vi "camera_capture.vi"(11 "dup Message Queue":refnum<queue>) -> ()   [LabVIEW 2017]
uses:
  UI Error Handlers/support/Message Queue/Message Cluster.ctl
  <vilib>/userdefined/High Color/IMAQdx.ctl
  <vilib>/vision/Avi.llb/IMAQ AVI2 Codec Path.ctl
  Globals/Global - All RT Loop Stop.vi
  <vilib>/vision/driver/NI_Vision_Acquisition_Software.lvlib
  UI Error Handlers/support/Message Queue/Message Queue.lvlib
panel:
  out "concatenated string 2":string
  in  "Boolean":bool
  out "Codec Names":string[](array[string])
  in  "stop":bool
  out "Webcam":T1(plugin-control)
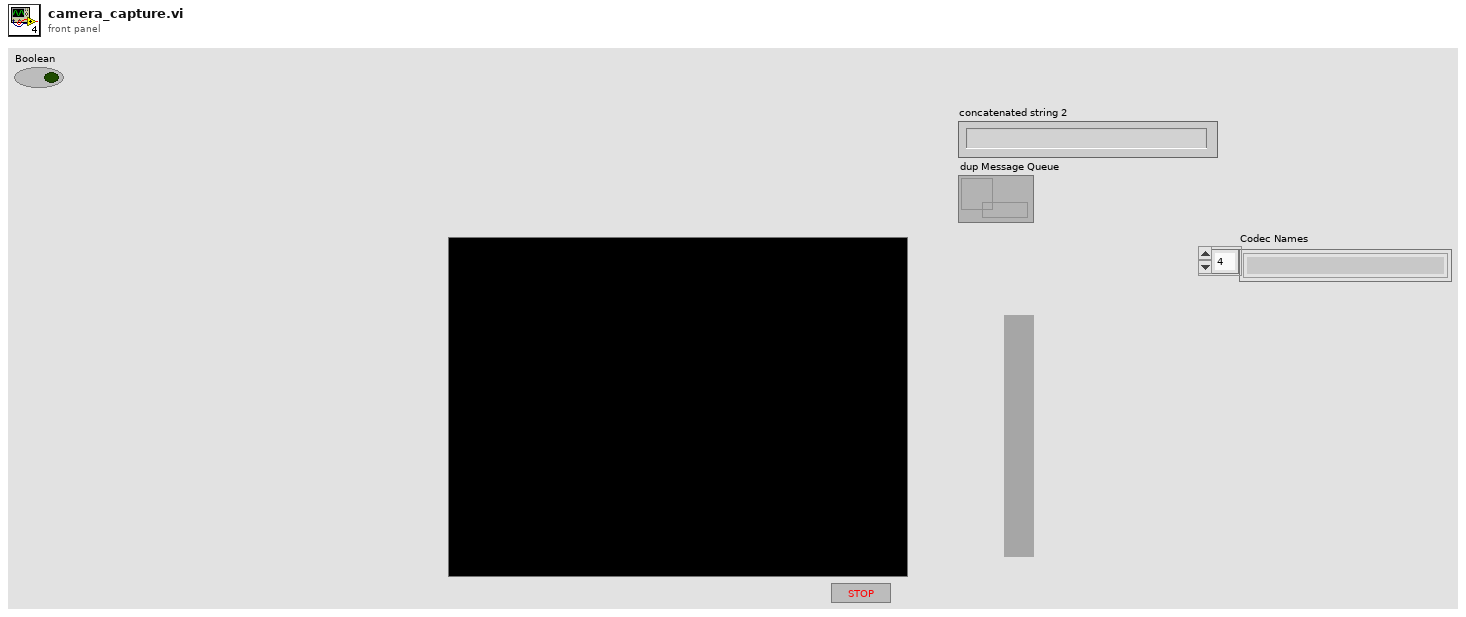
[diagram p1: front panel]
types:
  T1 = typedef "IMAQ Image.ctl" = refnum<image>
  T2 = typedef "IMAQdx.ctl" = refnum<k21>
  T3 = typedef "Image Type" = u32
  T4 = typedef "IMAQ AVI2 Refnum.ctl" = refnum<k20>
  T5 = typedef "IMAQ AVI2 Codec Path.ctl" = u32
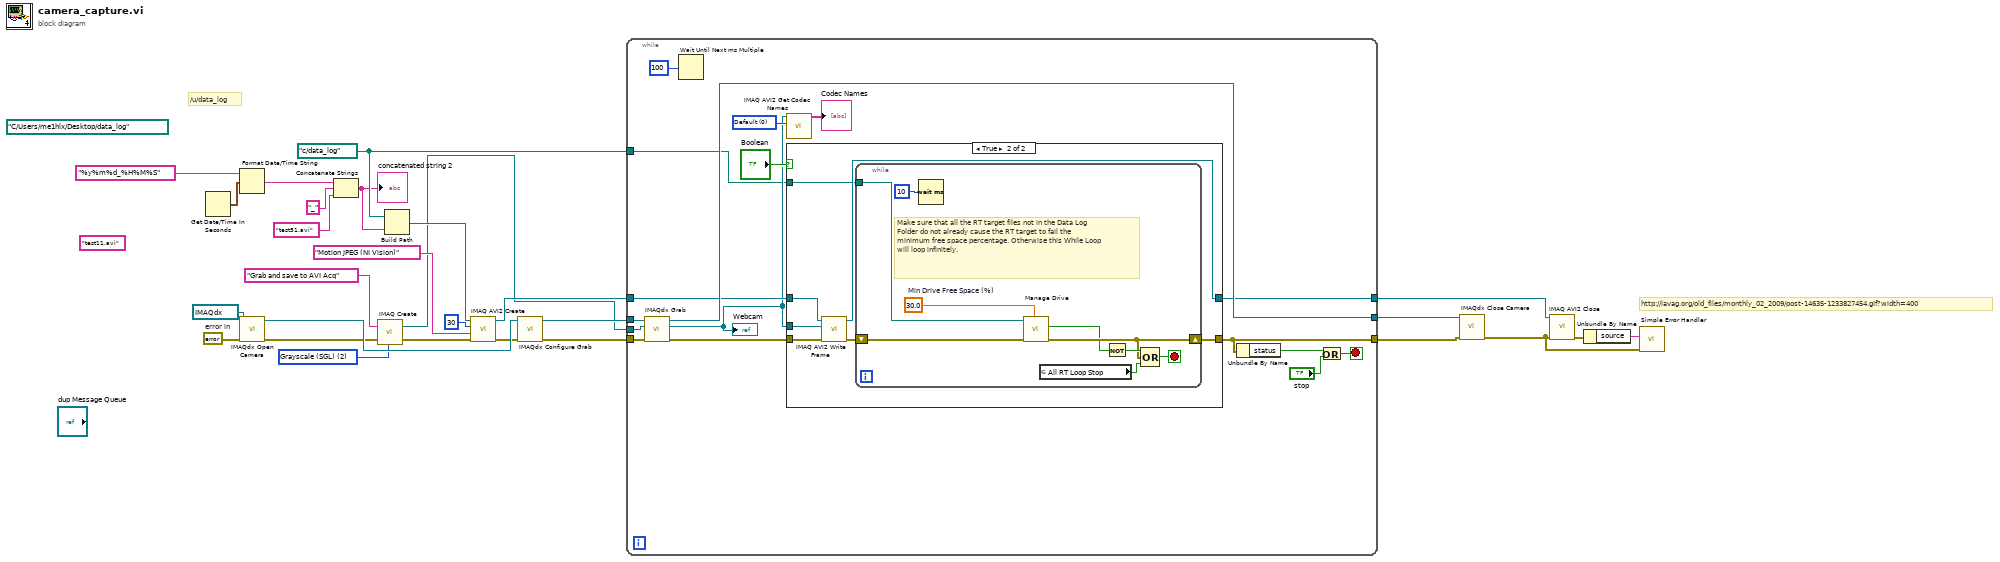
[diagram p0: block diagram]
diagram:
  (unwired) path "C:/Users/me1hlx/Desktop/data_log" ("AVI Path")
  (unwired) "test11.avi" ("name or relative path")
  w3 = path "c:/data_log" ("AVI Path")
  w17 = T3 2 items=["Grayscale (U8)", "Grayscale (I16)", "Grayscale (SGL)", "Complex (CSG)", "RGB (U32)", "HSL (U32)", "RGB (U64)", "Grayscale (U16)"] ("Image Type")
  w20 = errorcluster {"status"=FALSE, "code"=0, "source"=""}  # error in
  # "/u/data_log"
  # "http://lavag.org/old_files/monthly_02_2009/post-14635-1233827454.gif?width=400"
  n1 = Get Date/Time In Seconds() -> (seconds since 1Jan1904=w7:timestamp)
  n2 = Format Date/Time String(time format string (%c)="%y%m%d_%H%M%S", seconds (now)=w7) -> (date/time string=w6:string)  [unwired: 1 out]
  n3 = call <vilib>:"IMAQdx Open Camera.vi"("error in"=w20, "Session In"=T2 "cam0") -> ("error out"=w16:errorcluster, "Session Out"=w22:T2)  [unwired: 8 in]
  n4 = Concatenate Strings(w6, "_" ("string"), "test51.avi" ("name or relative path")) -> (w2:string)
  "concatenated string 2" <- w2
  n5 = call "IMAQ Create"("Image Name"="Grab and save to AVI Acq", "Image Type"=w17, "error in (no error)"=w16) -> ("New Image"=w9:T1, "error out"=w15:errorcluster)  [unwired: 2 in]
  n6 = Build Path(base path=w3, name or relative path=w2) -> (appended path=w19:path)
  n7 = call "IMAQ AVI2 Create"("error in (no error)"=w15, "Codec"="Motion JPEG (NI Vision)", "Frames Per Second"=u32 30, "AVI Path"=w19) -> ("error out"=w14:errorcluster, "AVI Refnum"=w12:T4)  [unwired: 6 in]
  n8 = call <vilib>:"IMAQdx Configure Grab.vi"("error in"=w14, "Session In"=w22) -> ("error out"=w10:errorcluster, "Session Out"=w11:T2)  [unwired: 8 in]
  n9 = while {
    tunnel: w10 -> [w45]
    tunnel: w11 -> [w44]
    tunnel: w9 -> [w43]
    tunnel: [w30] -> w28
    tunnel: [w42] -> w27
    tunnel: w12 -> [w34]
    tunnel: [w32] -> w23
    tunnel: w3 -> [w29]
    stop <- w38 stop-if-true
    w37 = T5 0 items=["Default", "System", "Built in Vision"] ("Codec Source")
    n10 = call <vilib>:"IMAQdx Grab.vi"("error in"=w45, "Image In"=w43, "Session In"=w44) -> ("error out"=w31:errorcluster, "Image Out"=w33:T1, "Session Out"=w42:T2)  [unwired: 5 in, 1 out]
    "Webcam" <- w33
    n11 = Wait Until Next ms Multiple(millisecond multiple=u32 100 ("milliseconds to wait")) -> ()  [unwired: 1 out]
    n12 = call "IMAQ AVI2 Get Codec Names"("Codec Source"=w37, "Image"=w33) -> ("Codec Names"=→"Codec Names":string[])  [unwired: 8 in, 1 out]
    n13 = case shown="True" "Boolean" {
      tunnel: w34 -> [w47 w54]
      tunnel: w33 -> [_ w53]
      tunnel: [w47 w52] -> w32
      tunnel: w31 -> [w46 w51]
      tunnel: [w46 w48] -> w30
      tunnel: w29 -> [_ w50]
      frame False {
      }
      frame True {
        n14 = call "IMAQ AVI2 Write Frame"("error in (no error)"=w51, "Image"=w53, "AVI Refnum"=w54) -> ("error out"=w49:errorcluster, "AVI Refnum (duplicate)"=w52:T4)  [unwired: 6 in, 1 out]
        n15 = while {
          shift-right: [w58] -> w48
          shift-left: w49 -> [w59]
          tunnel: w50 -> [w56]
          stop <- w63 stop-if-true
          w57 = 30.0  # Min Drive Free Space (%)
          # "Make sure that all the RT target files not in the Data Log Folder do not already cause the RT target to fail the minimum free space percentage. Otherwise this While Loop will loop infinitely."
          n16 = Wait (ms)(milliseconds to wait=u32 10) -> ()  [unwired: 1 out]
          n17 = call "Manage Drive.vi"("Min Drive Free Space (%)"=w57, "error in"=w59, "Data Folder"=w56) -> ("error out"=w58:errorcluster, "Drive Space Below Limit"=w55:bool)  [unwired: 6 in, 1 out]
          n18 = global read "Global - All RT Loop Stop.vi" "All RT Loop Stop"() -> (w60:bool)
          n19 = Not(x=w55) -> (.not. x?=w62:bool)
          n20 = Compound Arithmetic op=OR(w62, w58, w60) -> (w63:bool)
        }
      }
    }
    n21 = Unbundle By Name(w30) -> ("status"=w40:bool)
    n22 = Or(x=w40, y="stop") -> (x .or. y?=w38:bool)
  }
  n23 = call <vilib>:"IMAQdx Close Camera.vi"("error in"=w28, "Session In"=w27) -> ("error out"=w25:errorcluster)  [unwired: 9 in]
  n24 = call "IMAQ AVI2 Close"("error in (no error)"=w25, "AVI Refnum"=w23) -> ("error out"=w24:errorcluster)  [unwired: 9 in]
  n25 = Unbundle By Name(w24) -> ("source"=w26:string)
  n26 = call <vilib>:"Simple Error Handler.vi"("error source (\" \")"=w26, "error in (no error)"=w25) -> ()  [unwired: 3 in, 5 out]
